vi "Get Path Data.vi"(8 "error in":errorcluster, 11 "Path":path) -> (0 "error out":errorcluster, 3 "Path stuff":T1)   [LabVIEW 2019]
uses:
  Bordeaux/Command Stuff/Single Cmd Info.ctl
  <vilib>/picture/picture.llb/imagedata.ctl
  Bordeaux/Types/Limits.ctl
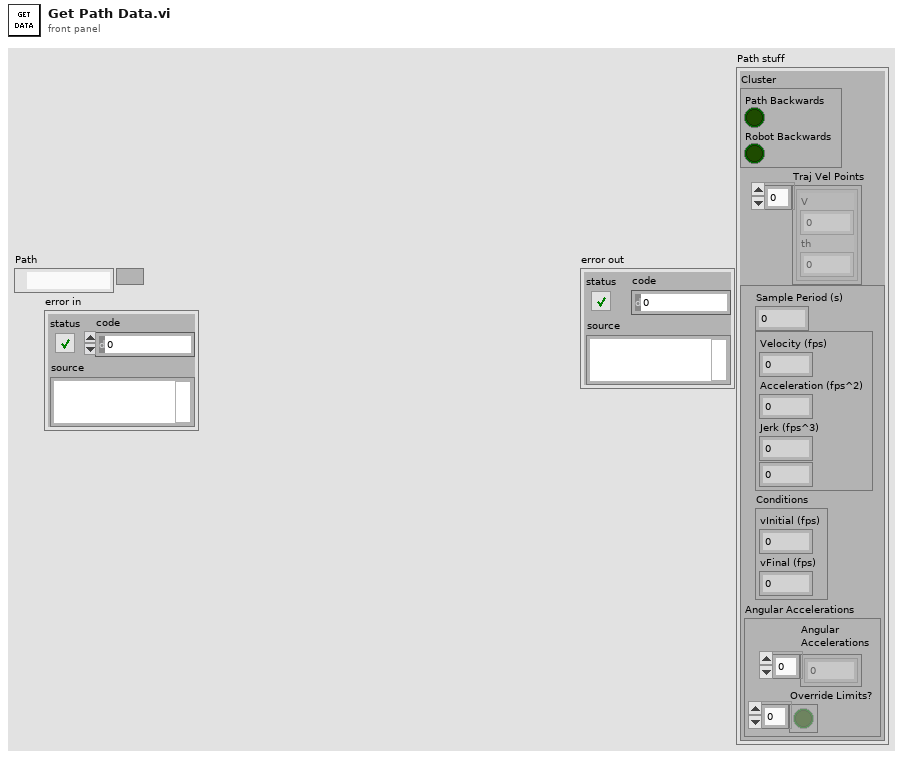
[diagram p1: front panel]
types:
  T1 = cluster{"Cluster":cluster{"Path Backwards":bool, "Robot Backwards":bool}, "Traj Vel Points":cluster{"V":dbl, "th":dbl}[], cluster{"Sample Period (s)":dbl, cluster{"Velocity (fps)":dbl, "Acceleration (fps^2)":dbl, "Jerk (fps^3)":dbl, dbl}, "Conditions":cluster{"vInitial (fps)":dbl, "vFinal (fps)":dbl}, "Angular Accelerations":cluster{"Angular \nAccelerations":dbl[], "Override Limits?":bool[]}}}
  T2 = cluster{"Segment Name":string, "Type":enum16{"Accel Straight", "Const Straight", "Blend", "Circle"}, "Traj Pos Points":cluster{"x":dbl, "y":dbl, "th":dbl}[], "Traj Vel Points":cluster{"V":dbl, "th":dbl}[], "Accel Index":i32, "Decel Index":i32}[]
  T3 = cluster{"Path Backwards":bool, "Robot Backwards":bool}
  T4 = typedef "Single Cmd Info.ctl" = cluster{"Name":string, "CPTM.DataType":variant, "All Control Values Variant":cluster{"Name":string, "Variant Data":variant}[], "icon full":T5, "icon scaled":T5, "Path":path, "Subsystem Color":u32}
  T5 = typedef "imagedata.ctl" = cluster{"image type":i32, "image depth":i32, "image":u8[], "mask":u8[], "colors":u32[], "Rectangle":cluster{"left":i16, "top":i16, "right":i16, "bottom":i16}}
  T6 = cluster{"Sample Period (s)":dbl, "Limits":cluster{"Velocity (fps)":dbl, "Acceleration (fps^2)":dbl, "Jerk (fps^3)":dbl}, "Conditions":cluster{"vInitial (fps)":dbl, "vFinal (fps)":dbl}, "Angular Accelerations":cluster{"Angular \nAccelerations":dbl[], "Override Limits?":bool[]}}
  T7 = typedef "Limits.ctl" = cluster{"Velocity (fps)":dbl, "Accel (fps^2)":dbl, "Jerk (fps^3)":dbl, "StoopidFast (fps)":dbl}
  T8 = cluster{"Sample Period (s)":dbl, "Limits":T7, "Conditions":cluster{"vInitial (fps)":dbl, "vFinal (fps)":dbl}, cluster{dbl[], bool[]}}
  T9 = cluster{"Reverse Path":bool, "Robot Backwards":bool}
  T10 = cluster{"Velocity (fps)":dbl, "Acceleration (fps^2)":dbl, "Jerk (fps^3)":dbl}
  T11 = cluster{"vInitial (fps)":dbl, "vFinal (fps)":dbl}
  T12 = cluster{"Angular \nAccelerations":dbl[], "Override Limits?":bool[]}
  T13 = cluster{"Velocity (fps)":dbl, "Acceleration (fps^2)":dbl, "Jerk (fps^3)":dbl, dbl}
  T14 = cluster{"Sample Period (s)":dbl, cluster{"Velocity (fps)":dbl, "Acceleration (fps^2)":dbl, "Jerk (fps^3)":dbl, dbl}, "Conditions":cluster{"vInitial (fps)":dbl, "vFinal (fps)":dbl}, "Angular Accelerations":cluster{"Angular \nAccelerations":dbl[], "Override Limits?":bool[]}}
  T15 = cluster{"output cluster":cluster{"Reverse Path":bool, "Robot Backwards":bool}, "Traj Vel Points":cluster{"V":dbl, "th":dbl}[], "output cluster":cluster{"Sample Period (s)":dbl, "Limits":T7, "Conditions":cluster{"vInitial (fps)":dbl, "vFinal (fps)":dbl}, cluster{dbl[], bool[]}}}
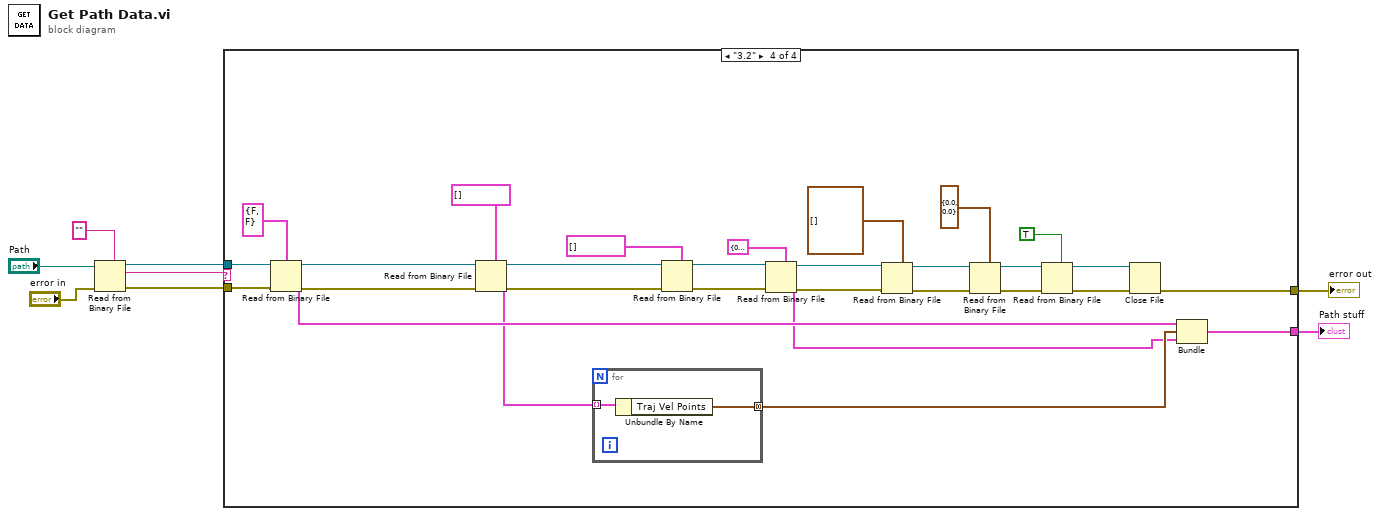
[diagram p0: block diagram]
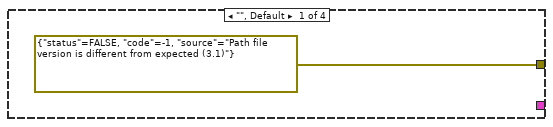
[diagram p2: hidden frame]
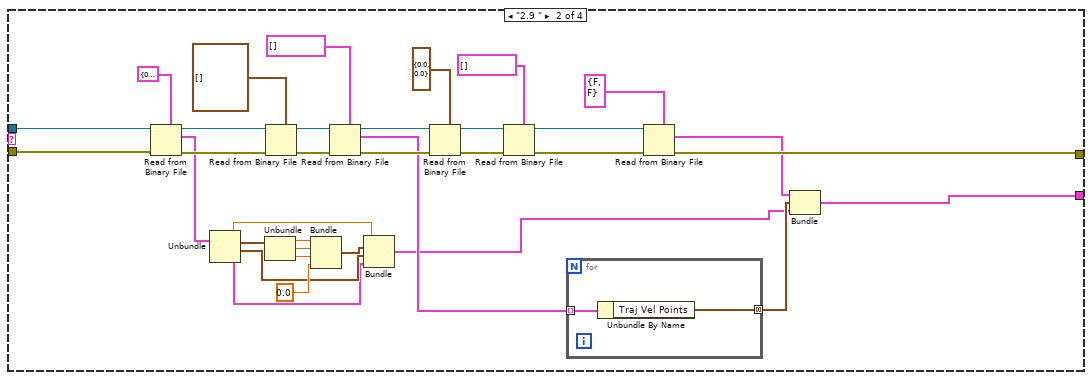
[diagram p3: hidden frame]
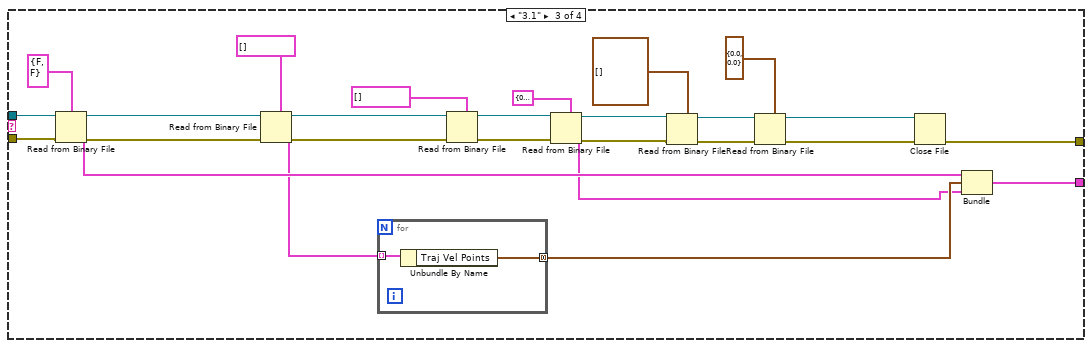
[diagram p4: hidden frame]
diagram:
  n1 = Read from Binary File(5:"", 8:"error in", 11:"Path") -> (0:w4:errorcluster, 2:w2:string, 3:w6:refnum<file>)  [unwired: 3 in, 1 out]
  n2 = case shown="\"3.2\"" w2 {
    tunnel: w6 -> [_ w36 w71 w102]
    tunnel: w4 -> [_ w31 w63 w94]
    tunnel: [errorcluster {"status"=FALSE, "code"=-1, "source"="Path file version is different from expected (3.1)"} ("error out") w25 w51 w84] -> w3
    tunnel: [_ w10 w47 w74] -> w1
    frame "", Default {
    }
    frame "2.9 " {
      n3 = Read from Binary File(5:T6 {"Sample Period (s)"=0.0, "Limits"={"Velocity (fps)"=0.0, "Acceleration (fps^2)"=0.0, "Jerk (fps^3)"=0.0}, "Conditions"={"vInitial (fps)"=0.0, "vFinal (fps)"=0.0}, "Angular Accelerations"={"Angular \nAccelerations"=[], "Override Limits?"=[]}}, 8:w31, 11:w36) -> (0:w30:errorcluster, 2:w21:T6, 3:w39:refnum<file>)  [unwired: 3 in, 1 out]
      n4 = Unbundle(w21) -> ("Sample Period (s)"=w15:dbl, "Limits"=w20:T10, "Conditions"=w13:T11, "Angular Accelerations"=w12:T12)
      n5 = Unbundle(w20) -> ("Velocity (fps)"=w19:dbl, "Acceleration (fps^2)"=w18:dbl, "Jerk (fps^3)"=w17:dbl)
      n6 = Read from Binary File(5:cluster{"x":dbl, "y":dbl, "th":dbl}[] [] ("Points"), 8:w30, 11:w39) -> (0:w29:errorcluster, 3:w40:refnum<file>)  [unwired: 3 in, 2 out]
      n7 = Bundle("Velocity (fps)"=w19, "Acceleration (fps^2)"=w18, "Jerk (fps^3)"=w17, 0.0) -> (w14:T13)  [unwired: 1 in]
      n8 = Read from Binary File(5:T2 [] ("Trajectory Data"), 8:w29, 11:w40) -> (0:w28:errorcluster, 2:w23:T2, 3:w41:refnum<file>)  [unwired: 3 in, 1 out]
      n9 = Bundle("Sample Period (s)"=w15, w14, "Conditions"=w13, "Angular Accelerations"=w12) -> (w11:T14)  [unwired: 1 in]
      n10 = Read from Binary File(5:cluster{"Time (s)":dbl, "Distance (ft)":dbl} {"Time (s)"=0.0, "Distance (ft)"=0.0}, 8:w28, 11:w41) -> (0:w27:errorcluster, 3:w42:refnum<file>)  [unwired: 3 in, 2 out]
      n11 = Read from Binary File(5:cluster{"Time (s)":dbl, T4, bool}[] [], 8:w27, 11:w42) -> (0:w26:errorcluster, 3:w43:refnum<file>)  [unwired: 3 in, 2 out]
      n12 = for {
        tunnel: w23 -> [w45] mode=indexing
        tunnel: [w44] -> w22 mode=concatenating
        n13 = Unbundle By Name(w45) -> ("Traj Vel Points"=w44:cluster{"V":dbl, "th":dbl}[])
      }
      n14 = Read from Binary File(5:T3 {"Path Backwards"=FALSE, "Robot Backwards"=FALSE} ("Cluster"), 8:w26, 11:w43) -> (0:w25:errorcluster, 2:w24:T3)  [unwired: 3 in, 2 out]
      n15 = Bundle("Cluster"=w24, "Traj Vel Points"=w22, w11) -> (w10:T1)  [unwired: 1 in]
    }
    frame "3.1" {
      n16 = Read from Binary File(5:T9 {"Reverse Path"=FALSE, "Robot Backwards"=FALSE} ("output cluster"), 8:w63, 11:w71) -> (0:w62:errorcluster, 2:w50:T9, 3:w69:refnum<file>)  [unwired: 3 in, 1 out]
      n17 = Read from Binary File(5:T2 [] ("Trajectory Data"), 8:w62, 11:w69) -> (0:w61:errorcluster, 2:w49:T2, 3:w67:refnum<file>)  [unwired: 3 in, 1 out]
      n18 = for {
        tunnel: w49 -> [w73] mode=indexing
        tunnel: [w72] -> w48 mode=concatenating
        n19 = Unbundle By Name(w73) -> ("Traj Vel Points"=w72:cluster{"V":dbl, "th":dbl}[])
      }
      n20 = Read from Binary File(5:cluster{"Time (s)":dbl, T4, bool}[] [], 8:w61, 11:w67) -> (0:w60:errorcluster, 3:w65:refnum<file>)  [unwired: 3 in, 2 out]
      n21 = Read from Binary File(5:T8 {"Sample Period (s)"=0.0, "Limits"={"Velocity (fps)"=0.0, "Accel (fps^2)"=0.0, "Jerk (fps^3)"=0.0, "StoopidFast (fps)"=0.0}, "Conditions"={"vInitial (fps)"=0.0, "vFinal (fps)"=0.0}, {[], []}} ("output cluster"), 8:w60, 11:w65) -> (0:w56:errorcluster, 2:w46:T8, 3:w59:refnum<file>)  [unwired: 3 in, 1 out]
      n22 = Read from Binary File(5:cluster{"x":dbl, "y":dbl, "th":dbl}[] [] ("Updated Waypoints"), 8:w56, 11:w59) -> (0:w55:errorcluster, 3:w57:refnum<file>)  [unwired: 3 in, 2 out]
      n23 = Read from Binary File(5:cluster{"Time (s)":dbl, "Distance (ft)":dbl} {"Time (s)"=0.0, "Distance (ft)"=0.0}, 8:w55, 11:w57) -> (0:w52:errorcluster, 3:w53:refnum<file>)  [unwired: 3 in, 2 out]
      n24 = Close File(refnum=w53, error in=w52) -> (error out=w51:errorcluster)  [unwired: 1 out]
      n25 = Bundle("output cluster"=w50, "Traj Vel Points"=w48, "output cluster"=w46) -> (w47:T15)  [unwired: 1 in]
    }
    frame "3.2" {
      n26 = Read from Binary File(5:T9 {"Reverse Path"=FALSE, "Robot Backwards"=FALSE} ("output cluster"), 8:w94, 11:w102) -> (0:w93:errorcluster, 2:w83:T9, 3:w100:refnum<file>)  [unwired: 3 in, 1 out]
      n27 = Read from Binary File(5:T2 [] ("Trajectory Data"), 8:w93, 11:w100) -> (0:w92:errorcluster, 2:w82:T2, 3:w98:refnum<file>)  [unwired: 3 in, 1 out]
      n28 = for {
        tunnel: w82 -> [w104] mode=indexing
        tunnel: [w103] -> w81 mode=concatenating
        n29 = Unbundle By Name(w104) -> ("Traj Vel Points"=w103:cluster{"V":dbl, "th":dbl}[])
      }
      n30 = Read from Binary File(5:cluster{"Time (s)":dbl, T4, bool}[] [], 8:w92, 11:w98) -> (0:w91:errorcluster, 3:w96:refnum<file>)  [unwired: 3 in, 2 out]
      n31 = Read from Binary File(5:T8 {"Sample Period (s)"=0.0, "Limits"={"Velocity (fps)"=0.0, "Accel (fps^2)"=0.0, "Jerk (fps^3)"=0.0, "StoopidFast (fps)"=0.0}, "Conditions"={"vInitial (fps)"=0.0, "vFinal (fps)"=0.0}, {[], []}} ("output cluster"), 8:w91, 11:w96) -> (0:w87:errorcluster, 2:w75:T8, 3:w90:refnum<file>)  [unwired: 3 in, 1 out]
      n32 = Read from Binary File(5:cluster{"x":dbl, "y":dbl, "th":dbl}[] [] ("Updated Waypoints"), 8:w87, 11:w90) -> (0:w86:errorcluster, 3:w88:refnum<file>)  [unwired: 3 in, 2 out]
      n33 = Read from Binary File(5:cluster{"Time (s)":dbl, "Distance (ft)":dbl} {"Time (s)"=0.0, "Distance (ft)"=0.0}, 8:w86, 11:w88) -> (0:w79:errorcluster, 3:w80:refnum<file>)  [unwired: 3 in, 2 out]
      n34 = Read from Binary File(5:TRUE, 8:w79, 11:w80) -> (0:w77:errorcluster, 3:w78:refnum<file>)  [unwired: 3 in, 2 out]
      n35 = Close File(refnum=w78, error in=w77) -> (error out=w84:errorcluster)  [unwired: 1 out]
      n36 = Bundle("output cluster"=w83, "Traj Vel Points"=w81, "output cluster"=w75) -> (w74:T15)  [unwired: 1 in]
    }
  }
  "error out" <- w3
  "Path stuff" <- w1
